vi "Waveform Graph.vi"() -> ()   [LabVIEW 2025]
doc: "Demonstrates how to generate random data and display it in a waveform graph to show measurement data."
uses:
  <vilib>/numeric/Random Number (Range) DBL.vi
panel:
  out "Random Data Graph":dbl[](graph)
  in  "lower limit":dbl
  in  "upper limit":dbl
  in  "?":bool
  # "Sample example of generating random data in Waveform graphs"
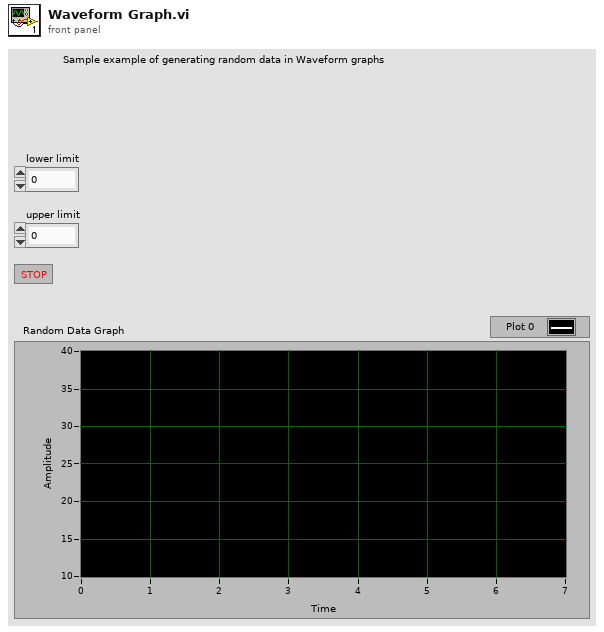
[diagram p1: front panel]
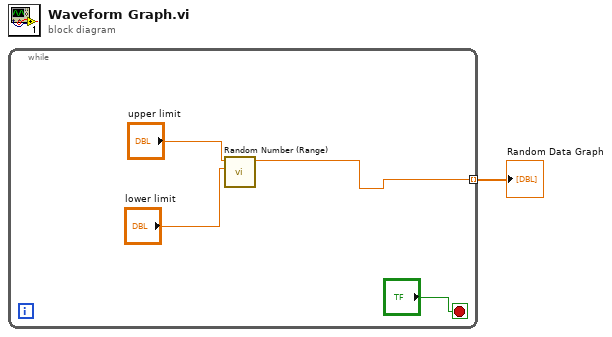
[diagram p0: block diagram]
diagram:
  n1 = while {
    tunnel: [w2] -> w1 mode=indexing
    stop <- "?" stop-if-true
    n2 = call-poly <vilib>:"Random Number (Range).vi"("lower bound (0)"="lower limit", "upper bound (100)"="upper limit") -> ("number"=w2:dbl)  [unwired: 9 in]
  }
  "Random Data Graph" <- w1
